vi "Revision Query Core.vi"(8 "error in (no error)":errorcluster, 11 "IVI_DMM_Delayed in":refnum<class "IVI_DMM_Delayed.lvclass">) -> (0 "error out":errorcluster, 1 "Firmware Revision":string, 2 "Driver Revision":string, 3 "IVI_DMM_Delayed out":refnum<class "IVI_DMM_Delayed.lvclass">)   [LabVIEW 2015, in "IVI_DMM.lvlib" / "IVI_DMM_Delayed.lvclass"]
uses:
  IVI_DMM_Delayed.lvclass
  IVI_DMM_Delayed.lvclass/IVI_DMM_Delayed.ctl
  IVI_DMM/IVI_DMM.lvclass
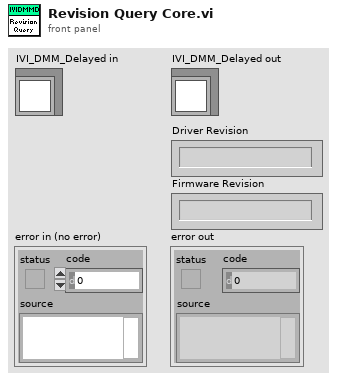
[diagram p1: front panel]
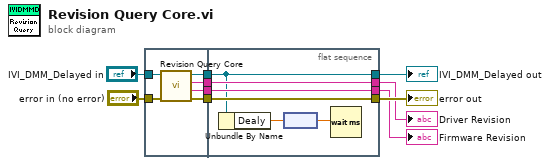
[diagram p0: block diagram]
diagram:
  n1 = flat-sequence {
    tunnel: "error in (no error)" -> [w12]
    tunnel: "IVI_DMM_Delayed in" -> [w11]
    tunnel: [w16] -> w4
    tunnel: [w15] -> w3
    tunnel: [w14] -> w2
    tunnel: [w13] -> w1
    tunnel: [w17] -> w7
    tunnel: [w20] -> w8
    tunnel: [w21] -> w9
    tunnel: [w22] -> w10
    tunnel: w4 -> [w22]
    tunnel: w3 -> [w21]
    tunnel: w2 -> [w20]
    tunnel: w1 -> [w17]
    frame #0 {
      n2 = call-parent "Revision Query Core.vi"("error in (no error)"=w12, "IVI_DMM in"=w11) -> ("error out"=w16:errorcluster, "Firmware Revision"=w15:string, "Driver Revision"=w14:string, "IVI_DMM out"=w13:refnum<class "IVI_DMM_Delayed.lvclass">)  [unwired: 6 in]
    }
    frame #1 {
      n3 = Unbundle By Name(w17) -> ("Dealy"=w18:dbl[unit])
      n4 = node(w18) -> (w19:dbl)
      n5 = Wait (ms)(milliseconds to wait=w19) -> ()  [unwired: 1 out]
    }
  }
  "error out" <- w10
  "IVI_DMM_Delayed out" <- w7
  "Driver Revision" <- w8
  "Firmware Revision" <- w9
